vi "Scenario Retrieve Record.vi"(8 "error in (no error)":errorcluster, 11 "Statement Refnum":T1) -> (0 "error out":errorcluster, 2 "Scenario":T2, 3 "Statement Refnum":T1)   [LabVIEW 2011]
uses:
  Scenario Record.ctl
  Conditions/Condition Record.ctl
  Conditions/Condition Operators.ctl
  SI.LIB/ODBC/SQL Controls/Statement Refnum.ctl
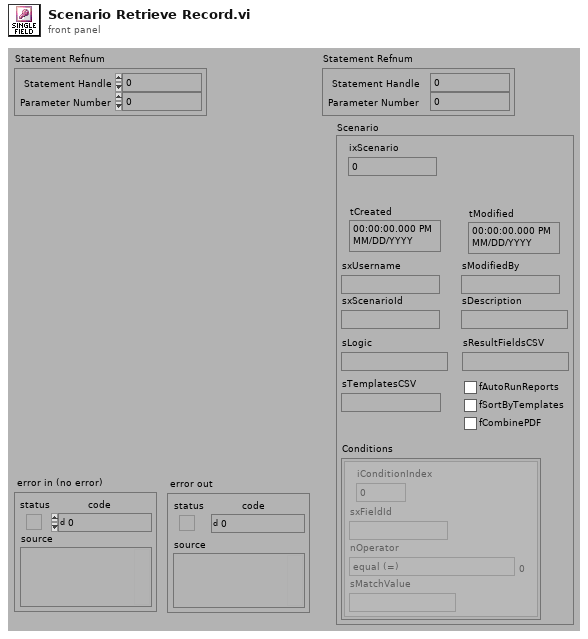
[diagram p1: front panel]
types:
  T1 = typedef "Statement Refnum.ctl" = cluster{"Statement Handle":i32, "Parameter Number":u16}
  T2 = typedef "Scenario Record.ctl" = cluster{"ixScenario":i32, "tCreated":timestamp, "tModified":timestamp, "sxUsername":string, "sModifiedBy":string, "sxScenarioId":string, "sDescription":string, "sLogic":string, "sResultFieldsCSV":string, "sTemplatesCSV":string, "fAutoRunReports":bool, "fSortByTemplates":bool, "fCombinePDF":bool, "Conditions":T3[]}
  T3 = typedef "Condition Record.ctl" = cluster{"iConditionIndex":i32, "sxFieldId":string, "nOperator":T4, "sMatchValue":string}
  T4 = typedef "Condition Operators.ctl" = enum16{"equal (=)", "not equal (\\u2260)", "less than (<)", "less than or equal (\\u2264)", "greater than (>)", "greater than or equal (\\u2265)", "contains", "does not contain"}
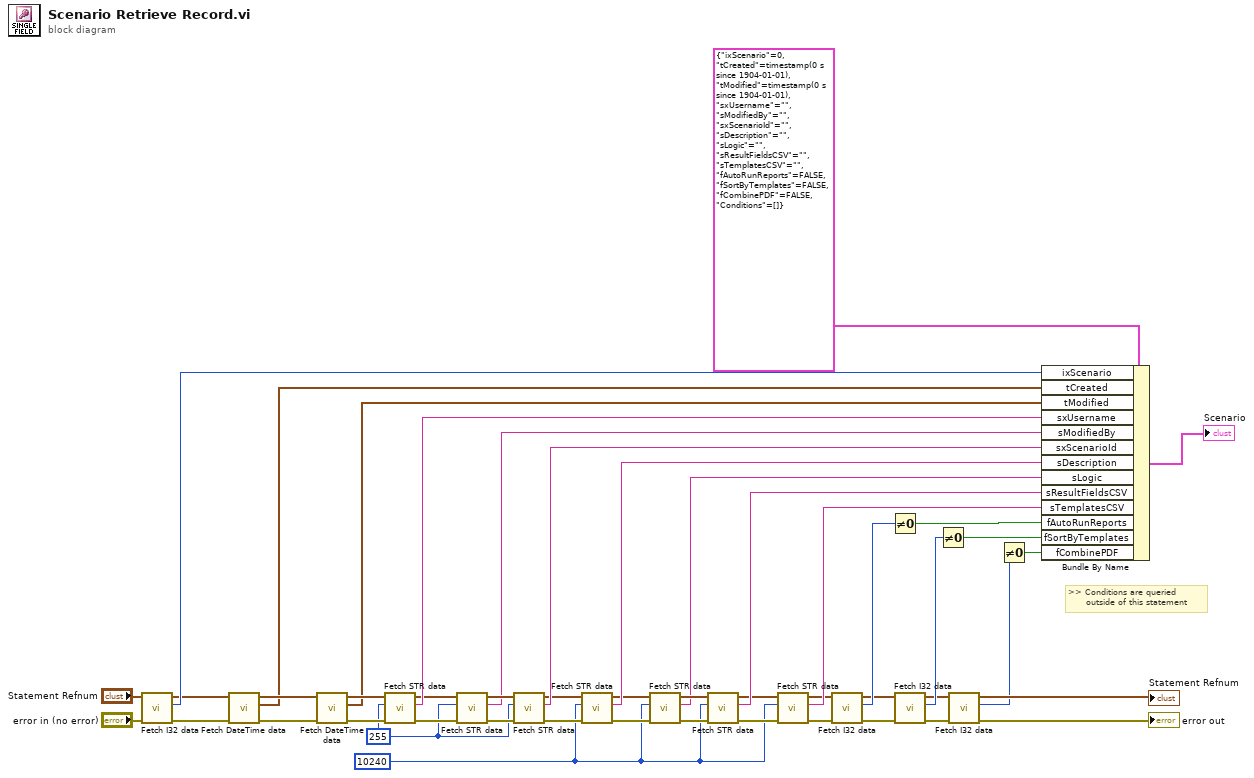
[diagram p0: block diagram]
diagram:
  w21 = 10240 ("Buffer Size")
  w26 = 255 ("Buffer Size")
  # ">> Conditions are queried\n      outside of this statement"
  n1 = call "Fetch I32 data.vi"("error in (no error)"="error in (no error)", "Statement Refnum"="Statement Refnum") -> ("error out"=w10:errorcluster, "Data"=w12:i32, "Statement Refnum"=w11:T1)  [unwired: 3 out]
  n2 = call "Fetch DateTime data.vi"("error in (no error)"=w10, "Statement Refnum"=w11) -> ("error out"=w9:errorcluster, "Data"=w7:timestamp, "Statement Refnum"=w8:T1)  [unwired: 3 out]
  n3 = call "Fetch DateTime data.vi"("error in (no error)"=w9, "Statement Refnum"=w8) -> ("error out"=w37:errorcluster, "Data"=w22:timestamp, "Statement Refnum"=w38:T1)  [unwired: 3 out]
  n4 = call "Fetch STR data.vi"("error in (no error)"=w37, "Buffer Size"=w26, "Statement Refnum"=w38) -> ("error out"=w29:errorcluster, "Data"=w44:string, "Statement Refnum"=w31:T1)  [unwired: 2 out]
  n5 = call "Fetch STR data.vi"("error in (no error)"=w29, "Buffer Size"=w26, "Statement Refnum"=w31) -> ("error out"=w28:errorcluster, "Data"=w27:string, "Statement Refnum"=w30:T1)  [unwired: 2 out]
  n6 = call "Fetch STR data.vi"("error in (no error)"=w28, "Buffer Size"=w26, "Statement Refnum"=w30) -> ("error out"=w35:errorcluster, "Data"=w46:string, "Statement Refnum"=w36:T1)  [unwired: 2 out]
  n7 = call "Fetch STR data.vi"("error in (no error)"=w35, "Buffer Size"=w21, "Statement Refnum"=w36) -> ("error out"=w33:errorcluster, "Data"=w34:string, "Statement Refnum"=w32:T1)  [unwired: 2 out]
  n8 = call "Fetch STR data.vi"("error in (no error)"=w33, "Buffer Size"=w21, "Statement Refnum"=w32) -> ("error out"=w41:errorcluster, "Data"=w40:string, "Statement Refnum"=w42:T1)  [unwired: 2 out]
  n9 = call "Fetch STR data.vi"("error in (no error)"=w41, "Buffer Size"=w21, "Statement Refnum"=w42) -> ("error out"=w24:errorcluster, "Data"=w39:string, "Statement Refnum"=w25:T1)  [unwired: 2 out]
  n10 = call "Fetch STR data.vi"("error in (no error)"=w24, "Buffer Size"=w21, "Statement Refnum"=w25) -> ("error out"=w5:errorcluster, "Data"=w23:string, "Statement Refnum"=w3:T1)  [unwired: 2 out]
  n11 = call "Fetch I32 data.vi"("error in (no error)"=w5, "Statement Refnum"=w3) -> ("error out"=w4:errorcluster, "Data"=w6:i32, "Statement Refnum"=w2:T1)  [unwired: 3 out]
  n12 = Not Equal To 0?(x=w6) -> (x != 0?=w1:bool)
  n13 = call "Fetch I32 data.vi"("error in (no error)"=w4, "Statement Refnum"=w2) -> ("error out"=w16:errorcluster, "Data"=w20:i32, "Statement Refnum"=w17:T1)  [unwired: 3 out]
  n14 = Not Equal To 0?(x=w20) -> (x != 0?=w19:bool)
  n15 = call "Fetch I32 data.vi"("error in (no error)"=w16, "Statement Refnum"=w17) -> ("error out"=→"error out":errorcluster, "Data"=w13:i32, "Statement Refnum"=→"Statement Refnum":T1)  [unwired: 3 out]
  n16 = Not Equal To 0?(x=w13) -> (x != 0?=w18:bool)
  n17 = Bundle By Name(cluster=T2 {"ixScenario"=0, "tCreated"=timestamp(0 s since 1904-01-01), "tModified"=timestamp(0 s since 1904-01-01), "sxUsername"="", "sModifiedBy"="", "sxScenarioId"="", "sDescription"="", "sLogic"="", "sResultFieldsCSV"="", "sTemplatesCSV"="", "fAutoRunReports"=FALSE, "fSortByTemplates"=FALSE, "fCombinePDF"=FALSE, "Conditions"=[]} ("Field Data Information"), "ixScenario"=w12, "tCreated"=w7, "tModified"=w22, "sxUsername"=w44, "sModifiedBy"=w27, "sxScenarioId"=w46, "sDescription"=w34, "sLogic"=w40, "sResultFieldsCSV"=w39, "sTemplatesCSV"=w23, "fAutoRunReports"=w1, "fSortByTemplates"=w19, "fCombinePDF"=w18) -> (→"Scenario":T2)
